vi "VariableManager_Reference.vi"(7 "Operation":enum16{"Get Tag", "Set Tag"}(ring), 8 "error in (no error)":errorcluster, 10 "Value":variant, 11 "Tag":string) -> (0 "error out":errorcluster, 2 "Value out":variant, 3 "Tag Out":string, 4 "Found":bool, 5 "All Tags":cluster{"Tags":string[], "Values":variant[]})   [LabVIEW 2021]
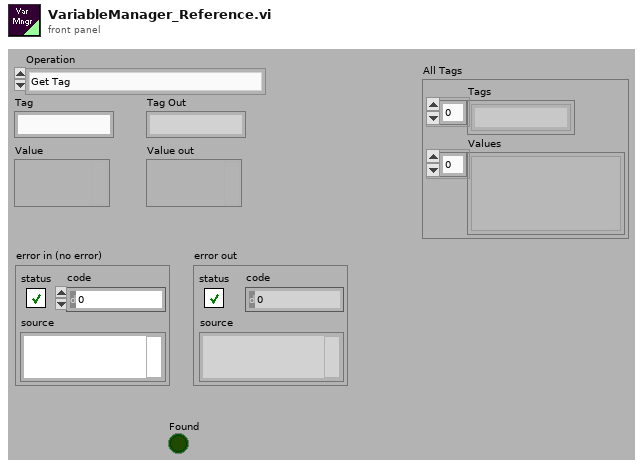
[diagram p1: front panel]
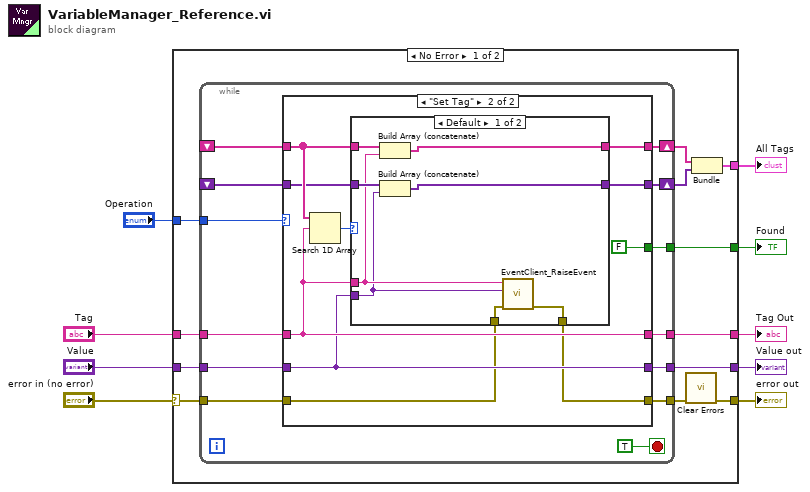
[diagram p0: block diagram]
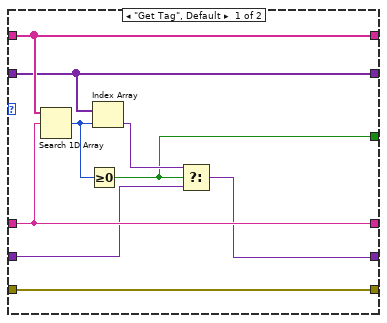
[diagram p2: hidden frame]
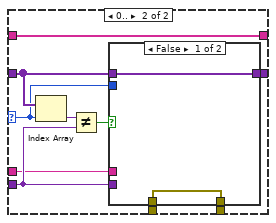
[diagram p3: hidden frame]
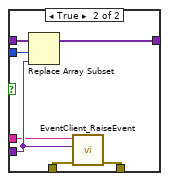
[diagram p4: hidden frame]
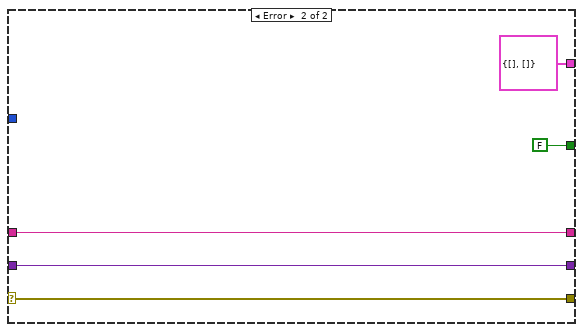
[diagram p5: hidden frame]
diagram:
  n1 = case shown="No Error" "error in (no error)" {
    selector: "error in (no error)" -> [w13 w83]
    tunnel: [w21 w85] -> w9
    tunnel: [w20 w84] -> w8
    tunnel: [w17 cluster{string[], variant[]} {[], []}] -> w7
    tunnel: [w10 w83] -> w6
    tunnel: "Tag" -> [w15 w85]
    tunnel: "Value" -> [w14 w84]
    tunnel: [w12 FALSE] -> w2
    tunnel: "Operation" -> [w11 _]
    frame No Error {
      n2 = while {
        shift-right: [w33] -> w19
        shift-left: _ -> [w34]
        shift-right: [w31] -> w18
        shift-left: _ -> [w32]
        tunnel: [w30] -> w21
        tunnel: [w29] -> w20
        tunnel: w13 -> [w27]
        tunnel: [w26] -> w16
        tunnel: w15 -> [w25]
        tunnel: w14 -> [w24]
        tunnel: [w23] -> w12
        tunnel: w11 -> [w22]
        stop <- TRUE stop-if-true
        n3 = case shown="\"Set Tag\"" w22 {
          tunnel: w34 -> [w43 w52]
          tunnel: [w43 w51] -> w33
          tunnel: w32 -> [w42 w49]
          tunnel: [w42 w50] -> w31
          tunnel: w25 -> [w41 w48]
          tunnel: w24 -> [w35 w47]
          tunnel: [w41 w48] -> w30
          tunnel: [w38 w47] -> w29
          tunnel: w27 -> [w37 w46]
          tunnel: [w37 w45] -> w26
          tunnel: [w36 FALSE] -> w23
          frame "Get Tag", Default {
            n4 = Search 1D Array(1D array=w43, element=w41) -> (index of element=w40:i32)  [unwired: 1 out]
            n5 = Greater Or Equal To 0?(x=w40) -> (x >= 0?=w36:bool)
            n6 = Index Array(array=w42, index=w40) -> (element=w39:variant)
            n7 = Select(t=w39, s=w36, f=w35) -> (s? t:f=w38:variant)
          }
          frame "Set Tag" {
            n8 = Search 1D Array(1D array=w52, element=w48) -> (index of element=w53:i32)  [unwired: 1 out]
            n9 = case shown="Default" w53 {
              selector: w53 -> [_ w66]
              tunnel: [w60 w71] -> w51
              tunnel: w52 -> [w61 w71]
              tunnel: [w58 w67] -> w50
              tunnel: w49 -> [w59 w68]
              tunnel: w48 -> [w55 w64]
              tunnel: w47 -> [w54 w65]
              tunnel: w46 -> [w57 w63]
              tunnel: [w56 w62] -> w45
              frame Default {
                n10 = Build Array (concatenate)(w61, w55) -> (w60:string[])
                n11 = Build Array (concatenate)(w59, w54) -> (w58:variant[])
                n12 = call "EventClient_RaiseEvent.vi"("error in (no error)"=w57, "Data"=w54, "Event"=w55) -> ("error out"=w56:errorcluster)  [unwired: 1 in, 7 out]
              }
              frame 0.. {
                n13 = Index Array(array=w68, index=w66) -> (element=w70:variant)
                n14 = Not Equal?(x=w70, y=w65) -> (x != y?=w69:bool)
                n15 = case shown="False" w69 {
                  tunnel: w68 -> [w73 w80]
                  tunnel: [w73 w79] -> w67
                  tunnel: w66 -> [_ w78]
                  tunnel: w65 -> [_ w76]
                  tunnel: w64 -> [_ w75]
                  tunnel: w63 -> [w72 w77]
                  tunnel: [w72 w74] -> w62
                  frame False {
                  }
                  frame True {
                    n16 = Replace Array Subset(array=w80, new element=w76, index=w78) -> (w79:variant[])
                    n17 = call "EventClient_RaiseEvent.vi"("error in (no error)"=w77, "Data"=w76, "Event"=w75) -> ("error out"=w74:errorcluster)  [unwired: 1 in, 7 out]
                  }
                }
              }
            }
          }
        }
      }
      n18 = call <vilib>:"Clear Errors.vi"("error in (no error)"=w16) -> ("error out"=w10:errorcluster)  [unwired: 5 in, 1 out]
      n19 = Bundle(w19, w18) -> (w17:cluster{string[], variant[]})  [unwired: 1 out]
    }
    frame Error {
    }
  }
  "Tag Out" <- w9
  "Value out" <- w8
  "All Tags" <- w7
  "error out" <- w6
  "Found" <- w2
